vi "A_6_inaczej.vi"() -> ()   [LabVIEW 2020]
panel:
  out "Time in sec 2":dbl format="%#_15g"
  out "First number 2":dbl
  out "Second number 2":dbl
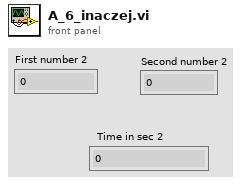
[diagram p1: front panel]
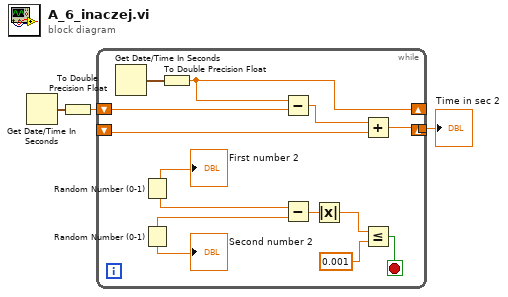
[diagram p0: block diagram]
diagram:
  n1 = Get Date/Time In Seconds() -> (seconds since 1Jan1904=w3:timestamp)
  n2 = To Double Precision Float(number=w3) -> (double precision float=w2:dbl)
  n3 = while {
    shift-right: [w8] -> _
    shift-left: w2 -> [w9]
    shift-right: [w4] -> _
    shift-left: _ -> [w5]
    tunnel: [w4] -> w1
    stop <- w12 stop-if-true
    n4 = Get Date/Time In Seconds() -> (seconds since 1Jan1904=w7:timestamp)
    n5 = Random Number (0-1)() -> (number: 0 to 1=w11:dbl)
    "First number 2" <- w11
    n6 = Random Number (0-1)() -> (number: 0 to 1=w10:dbl)
    "Second number 2" <- w10
    n7 = To Double Precision Float(number=w7) -> (double precision float=w8:dbl)
    n8 = Subtract(x=w8, y=w9) -> (x-y=w6:dbl)
    n9 = Subtract(x=w11, y=w10) -> (x-y=w15:dbl)
    n10 = Absolute Value(x=w15) -> (abs(x)=w14:dbl)
    n11 = Add(x=w6, y=w5) -> (x+y=w4:dbl)
    n12 = Less Or Equal?(x=w14, y=0.001) -> (x <= y?=w12:bool)
  }
  "Time in sec 2" <- w1
